vi "color clusters.vi"() -> ()   [LabVIEW 2013]
panel:
  out "Array":dbl[][][](array[numeric])
  in  "Weighted array of NEW cluster centers":dbl[][][](array[numeric])
  out "Array 2":u32[][][](array[colorbox])=[[[16448250, 6878717, 243648, 2448086, 215036, 7470158, 1425154, 15857665, 16566787, 16714500, 9895940]]]
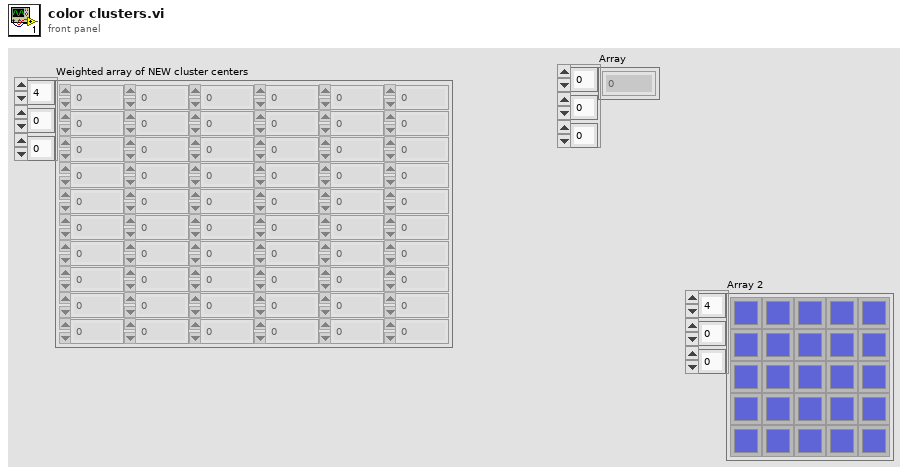
[diagram p1: front panel]
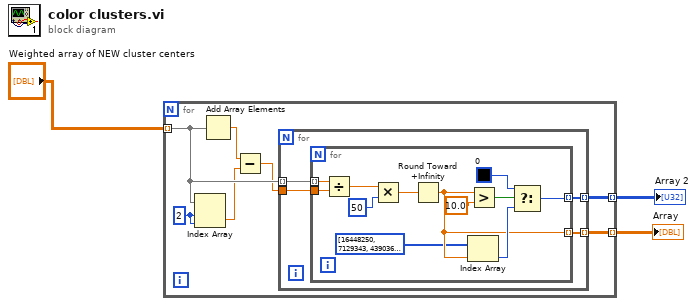
[diagram p0: block diagram]
diagram:
  n1 = for {
    tunnel: "Weighted array of NEW cluster centers" -> [w10] mode=indexing
    tunnel: [w5] -> w3 mode=indexing
    tunnel: [w4] -> w1 mode=indexing
    w9 = 2 ("index (row)")
    n2 = Index Array(array=w10, index (row)=w9, index (col)=w9) -> (element=w8:dbl)
    n3 = Add Array Elements(numeric array=w10) -> (sum=w7:dbl)
    n4 = Subtract(x=w7, y=w8) -> (x-y=w6:dbl)
    n5 = for {
      tunnel: w10 -> [w14] mode=indexing
      tunnel: w6 -> [w13]
      tunnel: [w12] -> w4 mode=indexing
      tunnel: [w11] -> w5 mode=indexing
      n6 = for {
        tunnel: w14 -> [w26] mode=indexing
        tunnel: w13 -> [w25]
        tunnel: [w16] -> w12 mode=indexing
        tunnel: [w17] -> w11 mode=indexing
        n7 = Divide(x=w26, y=w25) -> (x/y=w24:dbl)
        n8 = Multiply(x=w24, y=50) -> (x*y=w22:dbl)
        n9 = Round Toward +Infinity(x=w22) -> (ceil(x): smallest int >= x=w16:dbl)
        n10 = Index Array(array=u32[] [16448250, 7129343, 4390369, 3473009, 720406, 10157357, 15137024, 16765472, 16350208, 16714500, 9895940] ("Array 2"), index=w16) -> (element=w18:u32)
        n11 = Greater?(x=w16, y=10.0) -> (0:w20:bool)
        n12 = Select(t=u32 0, s=w20, f=w18) -> (s? t:f=w17:u32)
      }
    }
  }
  "Array 2" <- w3
  "Array" <- w1
